vi "CleanUp.vi"(8 "error in (no error)":errorcluster, 11 "Prueba04 in":refnum<class "Prueba04.lvclass">) -> (0 "error out":errorcluster, 3 "Prueba04 out":refnum<class "Prueba04.lvclass">)   [LabVIEW 2019, in "Prueba04.lvclass"]
uses:
  Prueba04.lvclass
  C:/Users/ivan_/Documents/procal/Pruebas/Prueba/Prueba.lvclass
  Prueba/Prueba.lvclass/Prueba.ctl
  Prueba04.lvclass/Prueba04.ctl
  Base de Datos/SQLiteConnector/SQLiteConnection.lvclass
  Base de Datos/Base de Datos.lvclass
  Prueba/Prueba.lvclass
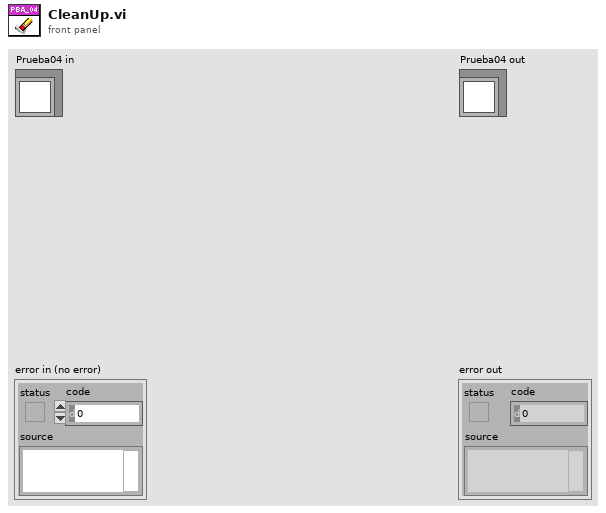
[diagram p1: front panel]
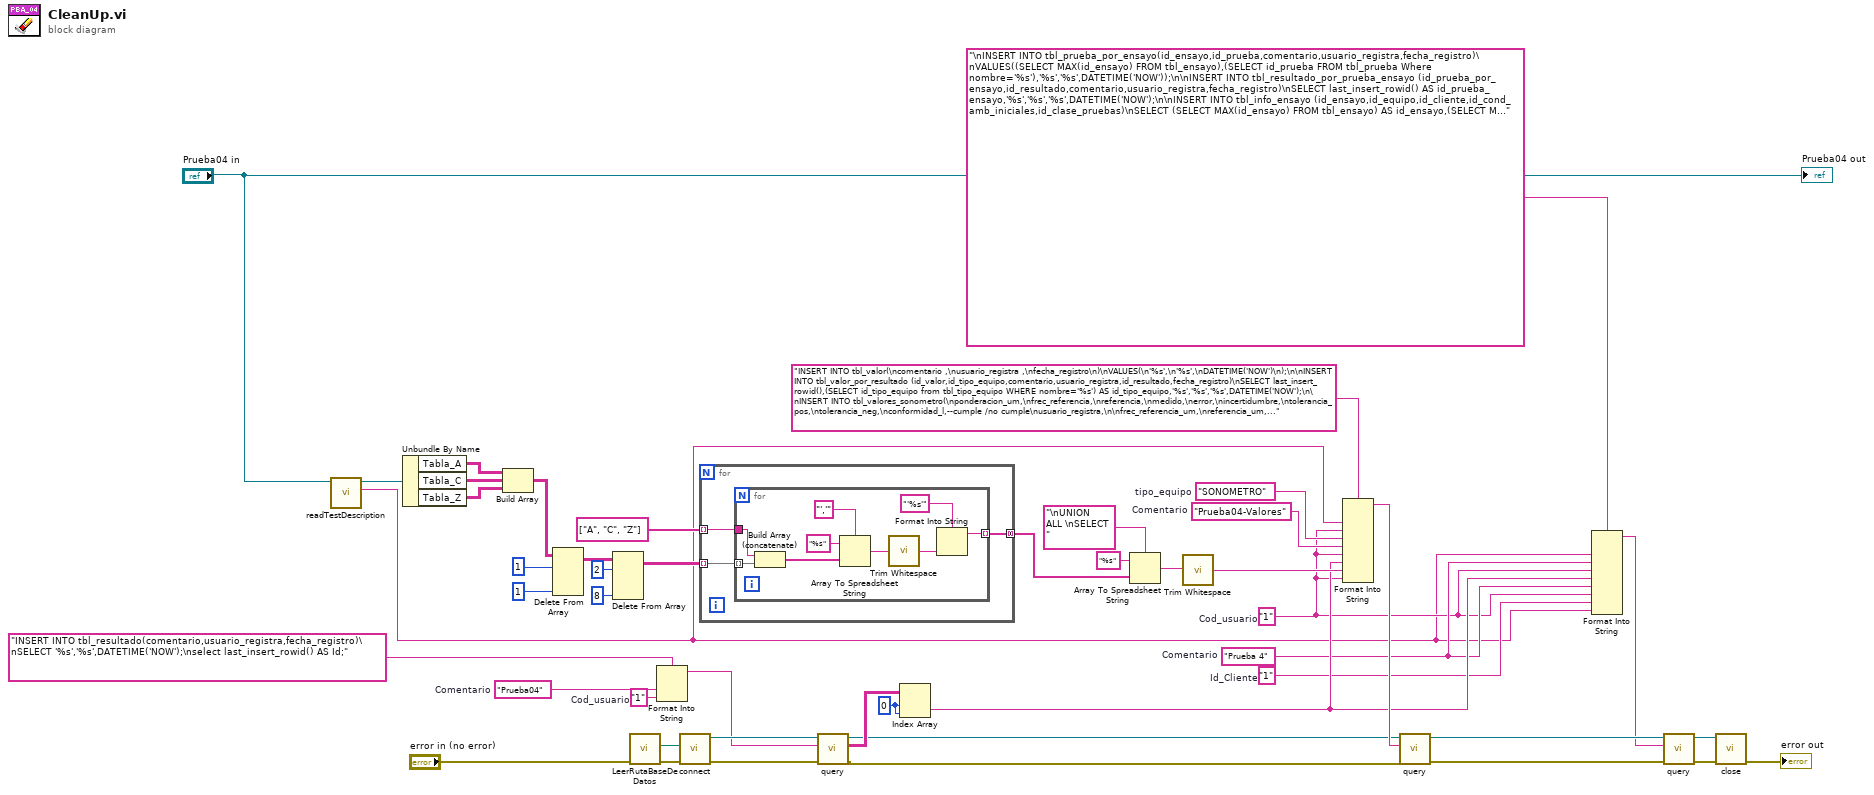
[diagram p0: block diagram]
diagram:
  w19 = "1"  # Id_Cliente
  w20 = "Prueba 4"  # Comentario
  w29 = "SONOMETRO"  # tipo_equipo
  w28 = "Prueba04-Valores"  # Comentario
  w34 = 0 ("index (row)")
  w36 = "1"  # Cod_usuario
  w37 = "Prueba04"  # Comentario
  w18 = "1"  # Cod_usuario
  n1 = call "readTestDescription.vi"("Prueba in"="Prueba04 in") -> ("Test Description"=w1:string, "Prueba out"=w2:refnum<class "Prueba04.lvclass">)  [unwired: 8 in, 1 out]
  n2 = Unbundle By Name(w2) -> ("Tabla_A"=w13:string[][], "Tabla_C"=w12:string[][], "Tabla_Z"=w11:string[][])
  n3 = Build Array(w13, w12, w11) -> (w9:string[][][])
  n4 = Delete From Array(array=w9, length=1, index (dim 2)=1 ("disabled index (col)")) -> (array with subset deleted=w7:string[][][])  [unwired: 2 in, 1 out]
  n5 = Delete From Array(array=w7, length=2, index (dim 2)=8 ("disabled index (col)")) -> (array with subset deleted=w16:string[][][])  [unwired: 2 in, 1 out]
  n6 = call "LeerRutaBaseDeDatos.vi"("error in (no error)"="error in (no error)") -> ("error out"=w42:errorcluster, "Database Path"=w41:path)  [unwired: 9 in]
  n7 = Format Into String(format string="INSERT INTO tbl_resultado(comentario,usuario_registra,fecha_registro)\nSELECT '%s','%s',DATETIME('NOW');\nselect last_insert_rowid() AS Id;" ("SQL Statement"), w37, w36) -> (resulting string=w35:string)  [unwired: 2 in, 1 out]
  n8 = call "connect.vi"("error in (no error)"=w42, "Database Path"=w41) -> ("error out"=w33:errorcluster, "object out"=w39:refnum<class "SQLiteConnection.lvclass">)  [unwired: 8 in]
  n9 = for {
    tunnel: [w50] -> w45 mode=concatenating
    tunnel: w16 -> [w49] mode=indexing
    tunnel: string[] ["A", "C", "Z"] -> [w48] mode=indexing
    n10 = for {
      tunnel: w49 -> [w53] mode=indexing
      tunnel: [w56] -> w50 mode=indexing
      tunnel: w48 -> [w52]
      n11 = Build Array (concatenate)(w52, w53) -> (w51:string[])
      n12 = Array To Spreadsheet String(delimiter (Tab)="','", array=w51, 3:"%s" ("format string")) -> (spreadsheet string=w55:string)
      n13 = call <vilib>:"Trim Whitespace.vi"("string"=w55) -> ("trimmed string"=w54:string)  [unwired: 1 in]
      n14 = Format Into String(format string="'%s'", w54) -> (resulting string=w56:string)  [unwired: 2 in, 1 out]
    }
  }
  n15 = call "query.vi"("error in (no error)"=w33, "SQL Statement"=w35, "object in"=w39) -> ("error out"=w4:errorcluster, "result"=w32:string[][], "object out"=w31:refnum<class "SQLiteConnection.lvclass">)  [unwired: 5 in, 1 out]
  n16 = Index Array(array=w32, index (row)=w34, index (col)=w34) -> (element=w21:string)
  n17 = Array To Spreadsheet String(delimiter (Tab)="\nUNION ALL \nSELECT ", array=w45, 3:"%s" ("format string")) -> (spreadsheet string=w44:string)
  n18 = call <vilib>:"Trim Whitespace.vi"("string"=w44) -> ("trimmed string"=w30:string)  [unwired: 1 in]
  n19 = Format Into String(format string="INSERT INTO tbl_valor(\ncomentario ,\nusuario_registra ,\nfecha_registro\n)\nVALUES(\n'%s',\n'%s',\nDATETIME('NOW')\n);\n\nINSERT INTO tbl_valor_por_resultado (id_valor,id_tipo_equipo,comentario,usuario_registra,id_resultado,fecha_registro)\nSELECT last_insert_rowid(),(SELECT id_tipo_equipo from tbl_tipo_equipo WHERE nombre='%s') AS id_tipo_equipo,'%s','%s','%s',DATETIME('NOW');\n\nINSERT INTO tbl_valores_sonometro(\nponderacion_um,\nfrec_referencia,\nreferencia,\nmedido,\nerror,\nincertidumbre,\ntolerancia_pos,\ntolerancia_neg,\nconformidad_l,--cumple /no cumple\nusuario_registra,\n\nfrec_referencia_um,\nreferencia_um,\nmedido_um,\nerror_um,\nincertidumbre_um,\ntolerancia_pos_um,\ntolerancia_neg_um,\n\nid_valor,\nfecha_registro\n)\nSELECT * FROM(\nSELECT %s\n) AS T\nINNER JOIN\n(SELECT %s AS usuario,'Hz','dB','dB','dB','dB','dB','dB',(SELECT MAX(id_valor) FROM tbl_valor) AS id_valor,DATETIME('NOW') fecha ) AS F;\n", w1, w18, w29, w28, w18, w21, w30, w18) -> (resulting string=w40:string)  [unwired: 2 in, 1 out]
  n20 = call "query.vi"("error in (no error)"=w4, "SQL Statement"=w40, "object in"=w31) -> ("error out"=w25:errorcluster, "object out"=w27:refnum<class "SQLiteConnection.lvclass">)  [unwired: 5 in, 2 out]
  n21 = Format Into String(format string="\nINSERT INTO tbl_prueba_por_ensayo(id_ensayo,id_prueba,comentario,usuario_registra,fecha_registro)\nVALUES((SELECT MAX(id_ensayo) FROM tbl_ensayo),(SELECT id_prueba FROM tbl_prueba Where nombre='%s'),'%s','%s',DATETIME('NOW'));\n\nINSERT INTO tbl_resultado_por_prueba_ensayo (id_prueba_por_ensayo,id_resultado,comentario,usuario_registra,fecha_registro)\nSELECT last_insert_rowid() AS id_prueba_ensayo,'%s','%s','%s',DATETIME('NOW');\n\nINSERT INTO tbl_info_ensayo (id_ensayo,id_equipo,id_cliente,id_cond_amb_iniciales,id_clase_pruebas)\nSELECT (SELECT MAX(id_ensayo) FROM tbl_ensayo) AS id_ensayo,(SELECT MAX(id_equipo) FROM tbl_equipo) AS id_equipo,'%s' AS id_cliente,(SELECT MAX(id_cond_amb_iniciales) FROM tbl_cond_amb_iniciales) AS id_cond_amb_iniciales,\n(SELECT id_clase_prueba FROM tbl_clase_prueba WHERE id_clase=(SELECT id_clase FROM tbl_equipo ORDER BY id_equipo DESC LIMIT 1)  AND id_prueba=(SELECT id_prueba FROM tbl_prueba Where nombre='%s')) AS id_clase_pruebas;\n", w1, w20, w18, w21, w20, w18, w19, w1) -> (resulting string=w22:string)  [unwired: 2 in, 1 out]
  n22 = call "query.vi"("error in (no error)"=w25, "SQL Statement"=w22, "object in"=w27) -> ("error out"=w24:errorcluster, "object out"=w26:refnum<class "SQLiteConnection.lvclass">)  [unwired: 5 in, 2 out]
  n23 = call-dynamic "close.vi"("error in (no error)"=w24, "object in"=w26) -> ("error out"=→"error out":errorcluster)  [unwired: 8 in, 1 out]
  "Prueba04 out" <- "Prueba04 in"
